vi "Pcre2MakeTables8.vi"(8 "error in":errorcluster) -> (0 "error out":errorcluster, 3 "pTable":u64 format="%.0x")   [LabVIEW 2021, in "libpcre2-8.lvlib"]
uses:
  libpcre2-8.lvlib
  libpcre2-8-x32.dll
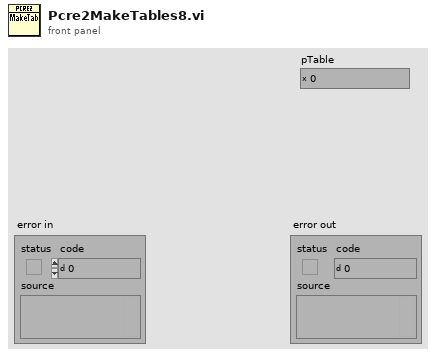
[diagram p1: front panel]
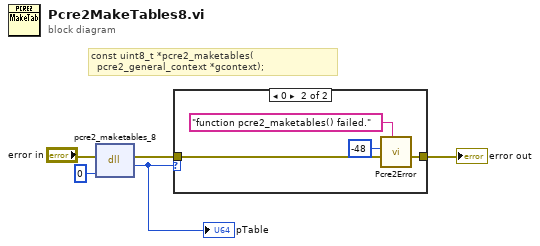
[diagram p0: block diagram]
diagram:
  # "const uint8_t *pcre2_maketables(\n  pcre2_general_context *gcontext);"
  n1 = dll-call lib="libpcre2-8-x*.dll" fn="pcre2_maketables_8"(error in="error in", "ctx"=u64 0) -> (error out=w3:errorcluster, "table"=w1:u64)  [unwired: 3 in, 1 out]
  "pTable" <- w1
  n2 = case shown="0" w1 {
    tunnel: w3 -> [w6 w9]
    tunnel: [w6 w8] -> w2
    frame Default {
    }
    frame 0 {
      n3 = call "Pcre2Error.vi"("message"="function pcre2_maketables() failed.", "error in"=w9, "ErrorCode"=-48) -> ("error out"=w8:errorcluster)  [unwired: 8 in]
    }
  }
  "error out" <- w2
